vi "UpAndDownDecimal.vi"() -> ()   [LabVIEW 2015]
panel:
  out "Number":dbl
  in  "Down Button":bool
  in  "Stop Button":bool
  out "bottom right":bool
  out "top right":bool
  out "bottom left":bool
  out "Top":bool
  out "Center":bool
  out "top left":bool
  out "Bottom":bool
  # "Count Up"
  # "Count Down"
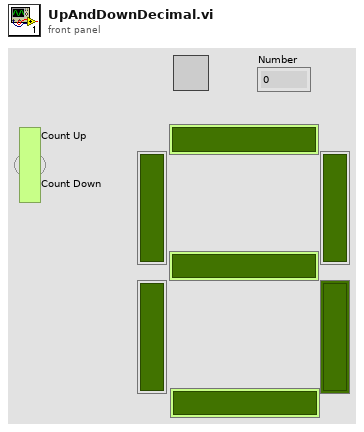
[diagram p1: front panel]
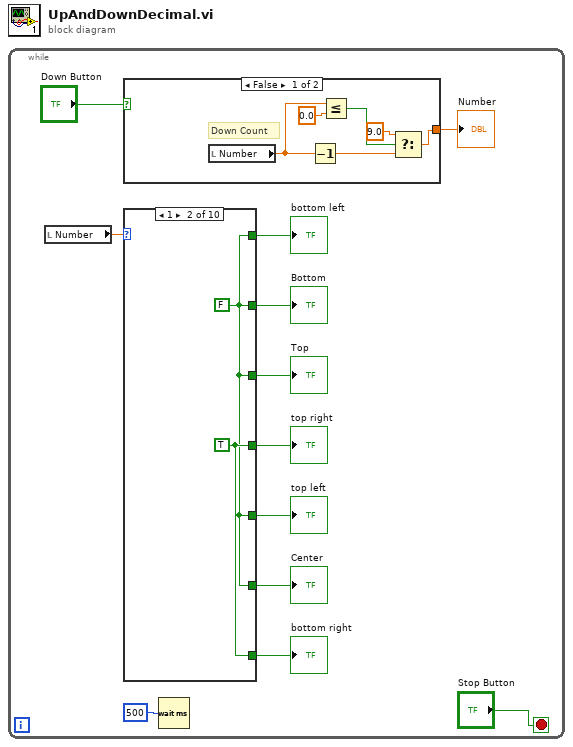
[diagram p0: block diagram]
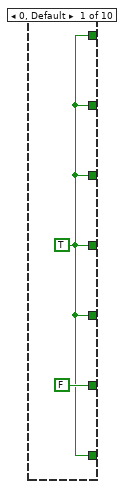
[diagram p2: hidden frame]
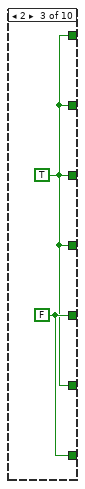
[diagram p3: hidden frame]
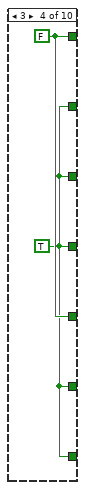
[diagram p4: hidden frame]
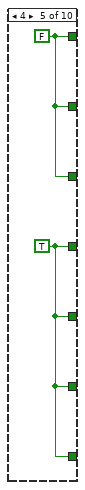
[diagram p5: hidden frame]
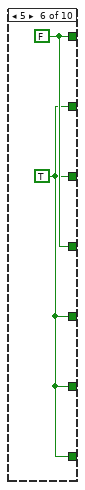
[diagram p6: hidden frame]
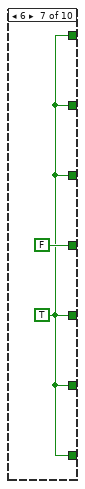
[diagram p7: hidden frame]
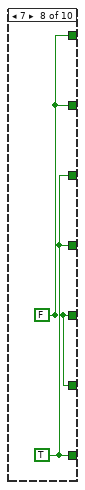
[diagram p8: hidden frame]
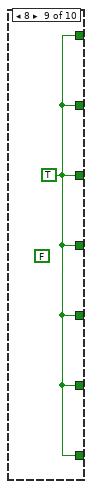
[diagram p9: hidden frame]
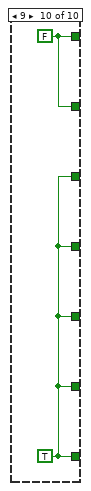
[diagram p10: hidden frame]
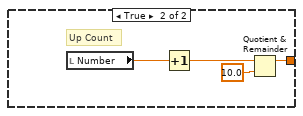
[diagram p11: hidden frame]
diagram:
  n1 = while {
    stop <- "Stop Button" stop-if-true
    n2 = local read "Number"() -> (w10:dbl)
    n3 = case shown="False" "Down Button" {
      tunnel: [w34 w39] -> w9
      frame False {
        # "Down Count"
        n4 = local read "Number"() -> (w33:dbl)
        n5 = Decrement(x=w33) -> (x-1=w32:dbl)
        n6 = Less Or Equal?(x=w33, y=0.0) -> (x <= y?=w36:bool)
        n7 = Select(t=9.0, s=w36, f=w32) -> (s? t:f=w34:dbl)
      }
      frame True {
        # "Up Count"
        n8 = local read "Number"() -> (w38:dbl)
        n9 = Increment(x=w38) -> (x+1=w40:dbl)
        n10 = Quotient & Remainder(x=w40, y=10.0 ("floor(x/y)")) -> (x-y*floor(x/y)=w39:dbl)  [unwired: 1 out]
      }
    }
    "Number" <- w9
    n11 = case shown="1" w10 {
      tunnel: [w13 w15 w17 w19 w22 w23 w25 w28 w29 w30] -> w7
      tunnel: [w13 w15 w18 w20 w21 w23 w25 w27 w29 w30] -> w6
      tunnel: [w13 w16 w17 w19 w21 w24 FALSE w28 w29 w30] -> w5
      tunnel: [FALSE w15 w17 w19 w21 w23 w25 w27 w29 w30] -> w4
      tunnel: [w13 w15 w17 w20 w22 w24 w25 w27 w29 w31] -> w3
      tunnel: [w13 w16 w18 w19 w21 w23 w25 w28 w29 w30] -> w2
      tunnel: [w13 w15 w17 w19 w22 w23 w25 w27 w29 w31] -> w1
      frame 0, Default {
        w13 = TRUE
      }
      frame 1 {
        w15 = FALSE
        w16 = TRUE
      }
      frame 2 {
        w18 = FALSE
        w17 = TRUE
      }
      frame 3 {
        w20 = FALSE
        w19 = TRUE
      }
      frame 4 {
        w22 = FALSE
        w21 = TRUE
      }
      frame 5 {
        w24 = FALSE
        w23 = TRUE
      }
      frame 6 {
        w25 = TRUE
      }
      frame 7 {
        w27 = FALSE
        w28 = TRUE
      }
      frame 8 {
        (unwired) FALSE
        w29 = TRUE
      }
      frame 9 {
        w31 = FALSE
        w30 = TRUE
      }
    }
    "Bottom" <- w1
    "top left" <- w6
    "Center" <- w4
    "Top" <- w7
    "bottom left" <- w3
    "top right" <- w5
    "bottom right" <- w2
    n12 = Wait (ms)(milliseconds to wait=u32 500 ("millisecond timer value")) -> ()  [unwired: 1 out]
  }
